vi "Enqueue.vi"(7 "EnqueType (Enque)":enum16{"LossyEnque", "EnqueAtFront", "Enque"}(ring), 8 "error in (no error)":errorcluster, 9 "Message Data":variant, 10 "Message":string, 11 "MessageQueue":refnum<queue>) -> (0 "error out":errorcluster, 3 "MessageQueue":refnum<queue>)   [LabVIEW 2018, in "AcPwrPlugins.lvlib"]
doc: "This VI adds an element to the queue. Each element is comprised of a message and data."
uses:
  AcPwrPlugins.lvlib
  clMessage.ctl
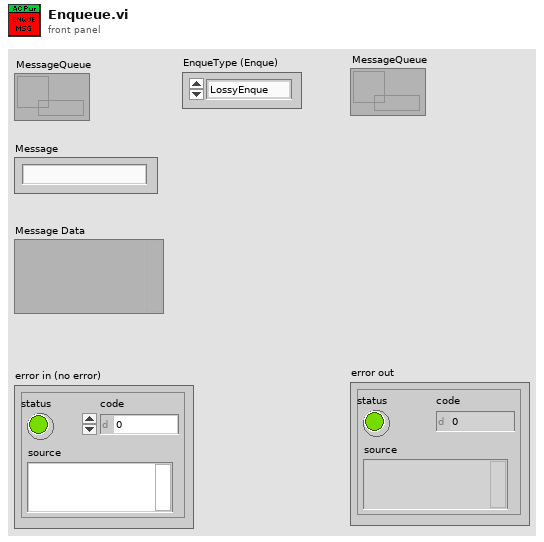
[diagram p1: front panel]
types:
  T1 = typedef "AcPwrPlugins.lvlib/clMessage.ctl" = cluster{"Message":string, "Message Data":variant}
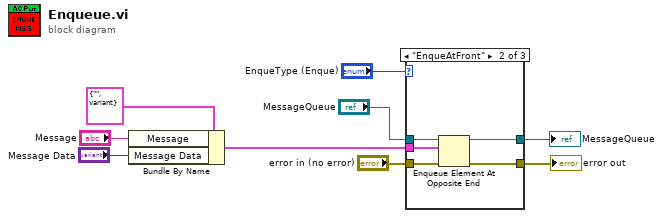
[diagram p0: block diagram]
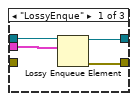
[diagram p2: hidden frame]
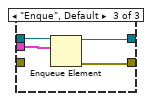
[diagram p3: hidden frame]
diagram:
  n1 = Bundle By Name(cluster=T1 {"Message"="", "Message Data"=variant} ("clMessage"), "Message"="Message", "Message Data"="Message Data") -> (w8:T1)
  n2 = case shown="\"EnqueAtFront\"" "EnqueType (Enque)" {
    tunnel: w8 -> [w10 w18 w21]
    tunnel: "MessageQueue" -> [w11 w17 w22]
    tunnel: [w12 w16 w19] -> w4
    tunnel: [w13 w15 w20] -> w2
    tunnel: "error in (no error)" -> [_ w14 _]
    frame "LossyEnque" {
      n3 = Lossy Enqueue Element(queue=w11, element=w10) -> (queue out=w12:refnum<queue>, error out=w13:errorcluster)  [unwired: 1 in, 2 out]
    }
    frame "EnqueAtFront" {
      n4 = Enqueue Element At Opposite End(queue=w17, element=w18, error in (no error)=w14) -> (queue out=w16:refnum<queue>, error out=w15:errorcluster)  [unwired: 1 in, 1 out]
    }
    frame "Enque", Default {
      n5 = Enqueue Element(queue=w22, element=w21) -> (queue out=w19:refnum<queue>, error out=w20:errorcluster)  [unwired: 2 in, 1 out]
    }
  }
  "error out" <- w2
  "MessageQueue" <- w4
